vi "subVI_CONEX_getPosition.vi"(3 "Error IN":errorcluster, 5 "CONEX Cluster":T1) -> (0 "error out":errorcluster, 1 "Current Position (mm)":dbl[](array[numeric]), 2 "CONEX Cluster out":T1)   [LabVIEW 2010]
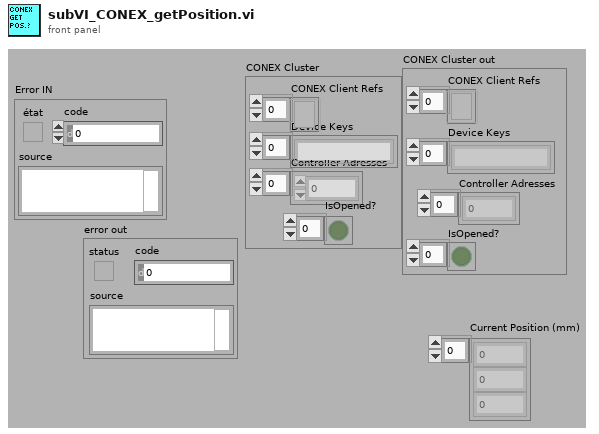
[diagram p1: front panel]
types:
  T1 = cluster{"CONEX Client Refs":refnum<k24>[], "Device Keys":string[], "Controller Adresses":i32[], "IsOpened?":bool[]}
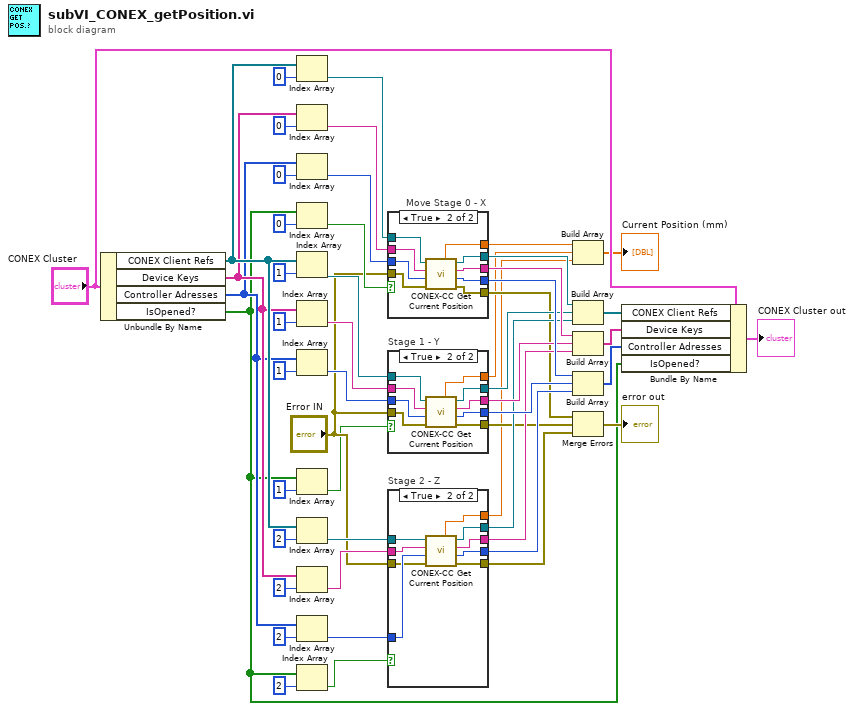
[diagram p0: block diagram]
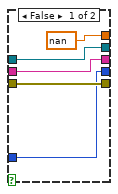
[diagram p2: hidden frame]
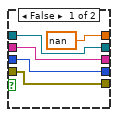
[diagram p3: hidden frame]
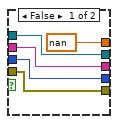
[diagram p4: hidden frame]
diagram:
  n1 = Unbundle By Name("CONEX Cluster") -> ("CONEX Client Refs"=w48:refnum<k24>[], "Device Keys"=w43:string[], "Controller Adresses"=w38:i32[], "IsOpened?"=w7:bool[])
  n2 = Index Array(array=w48, index=0) -> (element=w47:refnum<k24>)
  n3 = Index Array(array=w43, index=0) -> (element=w42:string)
  n4 = Index Array(array=w38, index=0) -> (element=w37:i32)
  n5 = Index Array(array=w7, index=0) -> (element=w28:bool)
  n6 = Index Array(array=w48, index=1) -> (element=w26:refnum<k24>)
  n7 = Index Array(array=w43, index=1) -> (element=w24:string)
  n8 = Index Array(array=w38, index=1) -> (element=w21:i32)
  n9 = Index Array(array=w7, index=1) -> (element=w5:bool)
  n10 = Index Array(array=w48, index=2) -> (element=w25:refnum<k24>)
  n11 = Index Array(array=w43, index=2) -> (element=w23:string)
  n12 = Index Array(array=w38, index=2) -> (element=w22:i32)
  n13 = Index Array(array=w7, index=2) -> (element=w8:bool)
  n14 = case "Move Stage 0 - X" shown="True" w28 {
    tunnel: w47 -> [w53 w65]
    tunnel: w42 -> [w54 w64]
    tunnel: w37 -> [w55 w63]
    tunnel: "Error IN" -> [w56 w62]
    tunnel: [w53 w61] -> w36
    tunnel: [w54 w60] -> w35
    tunnel: [w55 w59] -> w34
    tunnel: [w56 w58] -> w10
    tunnel: [nan ("Current position") w57] -> w4
    frame False {
    }
    frame True {
      n15 = call <userlib>:"CONEX-CC Get Current Position.vi"("CONEX Client Ref IN"=w65, "deviceKey IN"=w64, "Address IN"=w63, "Error IN"=w62) -> ("Current position"=w57:dbl, "CONEX Client Ref OUT"=w61:refnum<k24>, "deviceKey OUT"=w60:string, "Address OUT"=w59:i32, "Error OUT"=w58:errorcluster)
    }
  }
  n16 = case "Stage 1 - Y" shown="True" w5 {
    tunnel: w26 -> [w67 w79]
    tunnel: w24 -> [w68 w78]
    tunnel: w21 -> [w69 w77]
    tunnel: "Error IN" -> [w70 w76]
    tunnel: [w67 w75] -> w14
    tunnel: [w68 w74] -> w17
    tunnel: [w69 w73] -> w18
    tunnel: [w70 w72] -> w13
    tunnel: [nan ("Current position") w71] -> w3
    frame False {
    }
    frame True {
      n17 = call <userlib>:"CONEX-CC Get Current Position.vi"("CONEX Client Ref IN"=w79, "deviceKey IN"=w78, "Address IN"=w77, "Error IN"=w76) -> ("Current position"=w71:dbl, "CONEX Client Ref OUT"=w75:refnum<k24>, "deviceKey OUT"=w74:string, "Address OUT"=w73:i32, "Error OUT"=w72:errorcluster)
    }
  }
  n18 = case "Stage 2 - Z" shown="True" w8 {
    tunnel: w25 -> [w81 w93]
    tunnel: w23 -> [w82 w92]
    tunnel: w22 -> [w83 w91]
    tunnel: "Error IN" -> [w84 w90]
    tunnel: [w81 w89] -> w15
    tunnel: [w82 w88] -> w16
    tunnel: [w83 w87] -> w19
    tunnel: [w84 w86] -> w12
    tunnel: [nan ("Current position") w85] -> w2
    frame False {
    }
    frame True {
      n19 = call <userlib>:"CONEX-CC Get Current Position.vi"("CONEX Client Ref IN"=w93, "deviceKey IN"=w92, "Address IN"=w91, "Error IN"=w90) -> ("Current position"=w85:dbl, "CONEX Client Ref OUT"=w89:refnum<k24>, "deviceKey OUT"=w88:string, "Address OUT"=w87:i32, "Error OUT"=w86:errorcluster)
    }
  }
  n20 = Build Array(w4, w3, w2) -> (→"Current Position (mm)":dbl[])
  n21 = Build Array(w36, w14, w15) -> (w33:refnum<k24>[])
  n22 = Build Array(w35, w17, w16) -> (w32:string[])
  n23 = Build Array(w34, w18, w19) -> (w31:i32[])
  n24 = Merge Errors(w10, w13, w12) -> (→"error out":errorcluster)
  n25 = Bundle By Name(cluster="CONEX Cluster", "CONEX Client Refs"=w33, "Device Keys"=w32, "Controller Adresses"=w31, "IsOpened?"=w7) -> (→"CONEX Cluster out":T1)
